vi "CANOpen Export SDO.vi"(8 "error in (no error)":errorcluster, 10 "Display format":T2, 11 "SDO Parameters":T1[](array[typedef]) {"Sub-Index (0)" format="%.0x"; "Object Index" format="%.0x"; "Block Data" format="%.0x"}) -> (0 "error out":errorcluster)   [LabVIEW 2021, in "CANOpen Addon System Explorer.lvlib"]
uses:
  CANOpen Addon System Explorer.lvlib
  CANOpen_SDO data format.ctl
  Shared/CANOpen_SDO Settings.ctl
  Shared/CANOpen Addon Shared.lvlib
panel:
  out "spreadsheet string":string
  # "LSB"
  # "MSB"
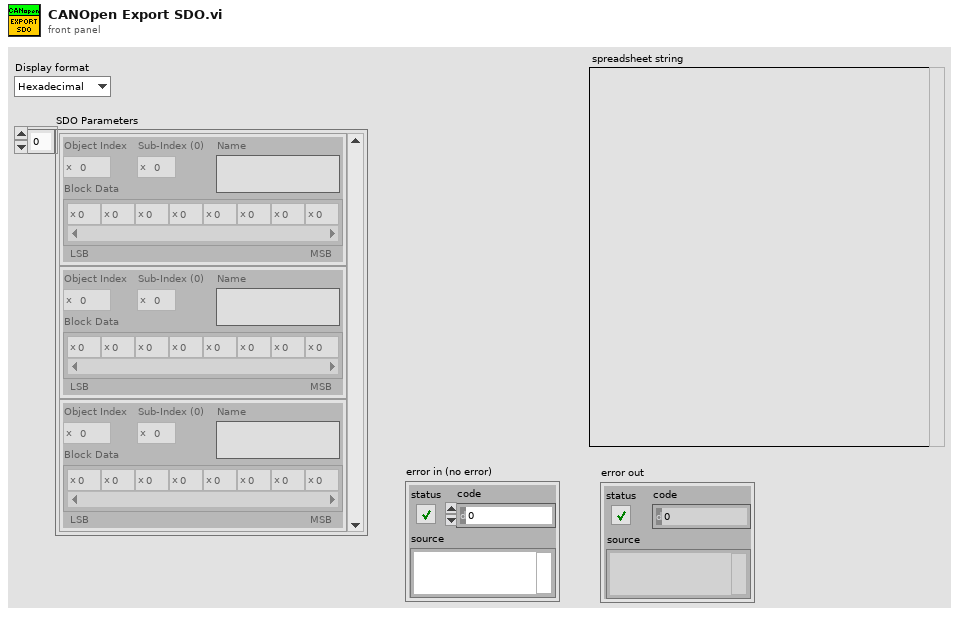
[diagram p1: front panel]
types:
  T1 = typedef "CANOpen Addon Shared.lvlib/CANOpen_SDO Settings.ctl" = cluster{"Object Index":u16, "Sub-Index (0)":u8, "Block Data":u8[], "Name":string}
  T2 = typedef "CANOpen Addon System Explorer.lvlib/CANOpen_SDO data format.ctl" = enum16{"Hexadecimal", "Decimal"}
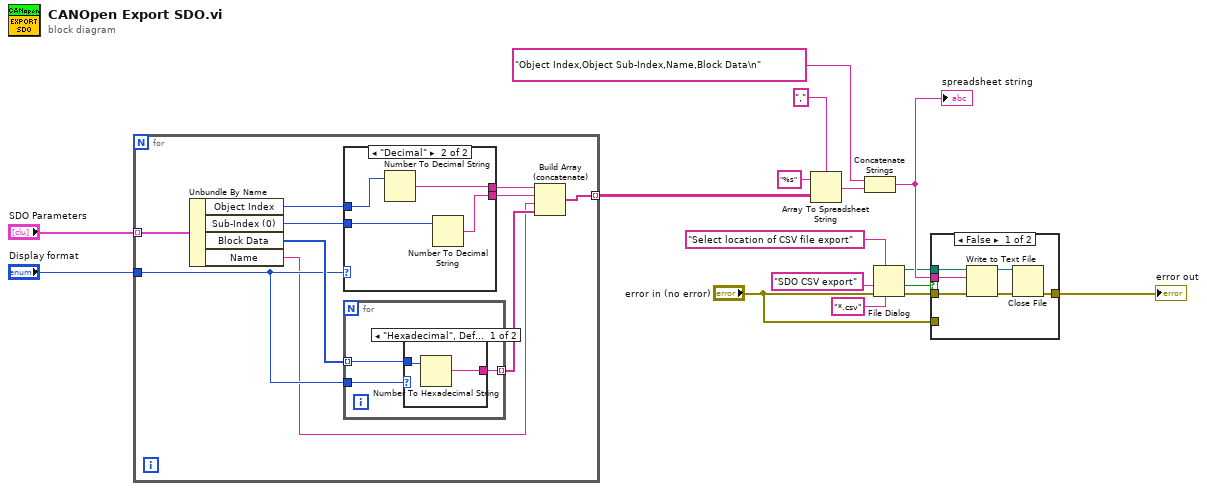
[diagram p0: block diagram]
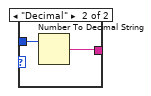
[diagram p3: hidden frame]
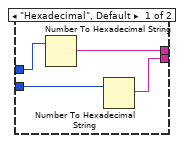
[diagram p4: hidden frame]
diagram:
  n1 = for {
    tunnel: "SDO Parameters" -> [w26] mode=indexing
    tunnel: "Display format" -> [w19]
    tunnel: [w21] -> w14 mode=indexing
    n2 = Unbundle By Name(w26) -> ("Object Index"=w25:u16, "Sub-Index (0)"=w22:u8, "Block Data"=w20:u8[], "Name"=w17:string)
    n3 = case shown="\"Decimal\"" w19 {
      tunnel: w25 -> [w37 w38]
      tunnel: [w36 w39] -> w24
      tunnel: [w35 w40] -> w23
      tunnel: w22 -> [w34 w41]
      frame "Hexadecimal", Default {
        n4 = Number To Hexadecimal String(2:w37) -> (0:w36:string)  [unwired: 1 in]
        n5 = Number To Hexadecimal String(2:w34) -> (0:w35:string)  [unwired: 1 in]
      }
      frame "Decimal" {
        n6 = Number To Decimal String(number=w38) -> (decimal integer string=w39:string)  [unwired: 1 in]
        n7 = Number To Decimal String(number=w41) -> (decimal integer string=w40:string)  [unwired: 1 in]
      }
    }
    n8 = for {
      tunnel: w20 -> [w29] mode=indexing
      tunnel: w19 -> [w28]
      tunnel: [w27] -> w18 mode=indexing
      n9 = case shown="\"Hexadecimal\", Default" w28 {
        tunnel: [w31 w33] -> w27
        tunnel: w29 -> [w30 w32]
        frame "Hexadecimal", Default {
          n10 = Number To Hexadecimal String(2:w30) -> (0:w31:string)  [unwired: 1 in]
        }
        frame "Decimal" {
          n11 = Number To Decimal String(number=w32) -> (decimal integer string=w33:string)  [unwired: 1 in]
        }
      }
    }
    n12 = Build Array (concatenate)(w24, w23, w17, w18) -> (w21:string[])
  }
  n13 = Array To Spreadsheet String(delimiter (Tab)=",", array=w14, 3:"%s" ("format string")) -> (spreadsheet string=w11:string)
  n14 = Concatenate Strings("Object Index,Object Sub-Index,Name,Block Data\n" ("string"), w11) -> (w2:string)
  "spreadsheet string" <- w2
  n15 = File Dialog(6:"*.csv" ("pattern (all files)"), 7:"Select location of CSV file export" ("prompt"), 8:"error in (no error)", 9:"SDO CSV export" ("default name")) -> (0:w5:errorcluster, 1:w6:bool, 3:w1:path)  [unwired: 3 in, 1 out]
  n16 = case shown="False" w6 {
    tunnel: w5 -> [w47 _]
    tunnel: [w42 w48] -> w4
    tunnel: "error in (no error)" -> [_ w48]
    tunnel: w2 -> [w46 _]
    tunnel: w1 -> [w45 _]
    frame False {
      n17 = Write to Text File(file (use dialog)=w45, text=w46, error in=w47) -> (refnum out=w43:refnum<file>, error out=w44:errorcluster)  [unwired: 1 in, 1 out]
      n18 = Close File(refnum=w43, error in=w44) -> (error out=w42:errorcluster)  [unwired: 1 out]
    }
    frame True {
    }
  }
  "error out" <- w4
